vi "msg(Reset).vi"   [LabVIEW 2014]
uses:
  <vilib>/FTP/NI_FTP.lvlib
types:
  T1 = typedef "NI_FTP.lvlib/FTP Session.ctl" = refnum<k5>
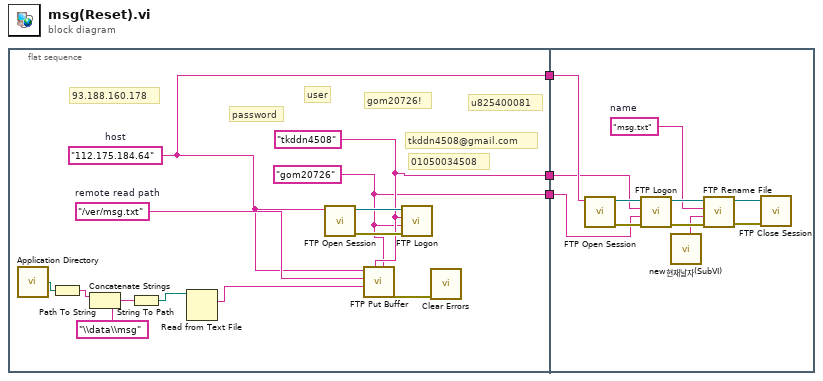
[diagram p0: block diagram]
diagram:
  n1 = flat-sequence {
    tunnel: [w6] -> w3
    tunnel: [w5] -> w2
    tunnel: [w4] -> w1
    tunnel: w3 -> [w27]
    tunnel: w2 -> [w20]
    tunnel: w1 -> [w19]
    frame #0 {
      w4 = "gom20726"
      w5 = "tkddn4508"
      w16 = "/ver/msg.txt"  # remote read path
      w6 = "112.175.184.64"  # host
      # "u825400081"
      # "93.188.160.178"
      # "gom20726!"
      # "01050034508"
      # "tkddn4508@gmail.com"
      # "user"
      # "password"
      n2 = call <vilib>:"Application Directory.vi"() -> ("Application Directory"=w13:path)
      n3 = Path To String(path=w13) -> (string=w11:string)
      n4 = Concatenate Strings(w11, "\\data\\msg" ("문자열")) -> (w10:string)
      n5 = String To Path(string=w10) -> (path=w9:path)
      n6 = Read from Text File(file (use dialog)=w9) -> (text=w8:string)  [unwired: 3 in, 3 out]
      n7 = call <vilib>:"FTP Open Session.vi"("address"=w6) -> ("error out"=w15:errorcluster, "ftp session"=w14:T1)  [unwired: 7 in, 2 out]
      n8 = call <vilib>:"FTP Put Buffer.vi"("password"=w4, "user"=w5, "data"=w8, "remote path"=w16, "host"=w6) -> ("error out"=w7:errorcluster)  [unwired: 5 in, 1 out]
      n9 = call <vilib>:"FTP Logon.vi"("error in (no error)"=w15, "password"=w4, "user"=w5, "ftp session"=w14) -> ()  [unwired: 4 in, 4 out]
      n10 = call <vilib>:"Clear Errors.vi"("error in (no error)"=w7) -> ()  [unwired: 5 in, 2 out]
    }
    frame #1 {
      w18 = "msg.txt"  # name
      n11 = call <vilib>:"FTP Open Session.vi"("address"=w27) -> ("error out"=w25:errorcluster, "ftp session"=w26:T1)  [unwired: 7 in, 2 out]
      n12 = call <vilib>:"FTP Logon.vi"("error in (no error)"=w25, "password"=w19, "user"=w20, "ftp session"=w26) -> ("error out"=w24:errorcluster, "ftp session out"=w23:T1)  [unwired: 4 in, 2 out]
      n13 = call "new현재날자(SubVI).vi"() -> ("날짜/시간 문자열"=w17:string)  [unwired: 5 in, 6 out]
      n14 = call <vilib>:"FTP Rename File.vi"("error in (no error)"=w24, "new name"=w17, "old name"=w18, "ftp session"=w23) -> ("error out"=w22:errorcluster, "ftp session out"=w21:T1)  [unwired: 4 in, 2 out]
      n15 = call <vilib>:"FTP Close Session.vi"("error in (no error)"=w22, "ftp session"=w21) -> ()  [unwired: 6 in, 4 out]
    }
  }
